vi "Configure Math.vi"(4 "dBm Resistance (600 Ohms)":i32(ring)=600 items=["50"=50, "75"=75, "93"=93, "110"=110, "124"=124, "125"=125, "135"=135, "150"=150, "250"=250, "300"=300, "500"=500, "600"=600, "800"=800, "900"=900, "1000"=1000, "1200"=1200, "8000"=8000], 5 "dB Reference (0.00 dBm)":dbl format="%.2f", 6 "Lower Limit (0.00)":dbl format="%.2f", 7 "Upper Limit (0.00)":dbl format="%.2f", 8 "error in (no error)":errorcluster, 9 "REL Offset (0.00)":dbl format="%_3f", 10 "Math Operation (0:None)":T1(ring), 11 "VISA resource name":refnum<visa-resource-name>) -> (0 "error out":errorcluster, 3 "VISA resource name out":refnum<visa-resource-name>)   [LabVIEW 2020, in "Library Instrument & Equipement.lvlib" / "Library Multimeter.lvlib" / "RIGOL DM3058.lvlib"]
doc: "Configures the Math Function on the instrument."
uses:
  RIGOL DM3058.lvlib
panel:
  # "Limit"
  # "DB Measurements"
  # "Offset"
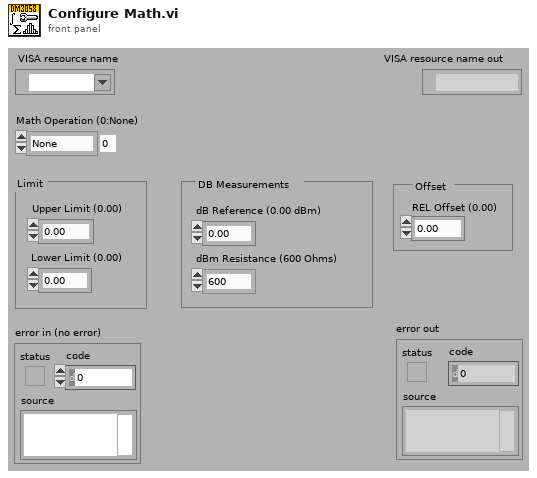
[diagram p1: front panel]
types:
  T1 = enum16{"None", "MAX", "MIN", "AVG", "P/F", "dB", "dBm", "REL"}
  T2 = cluster{"DM Series Mode":u16, "Measurement Function":u16}
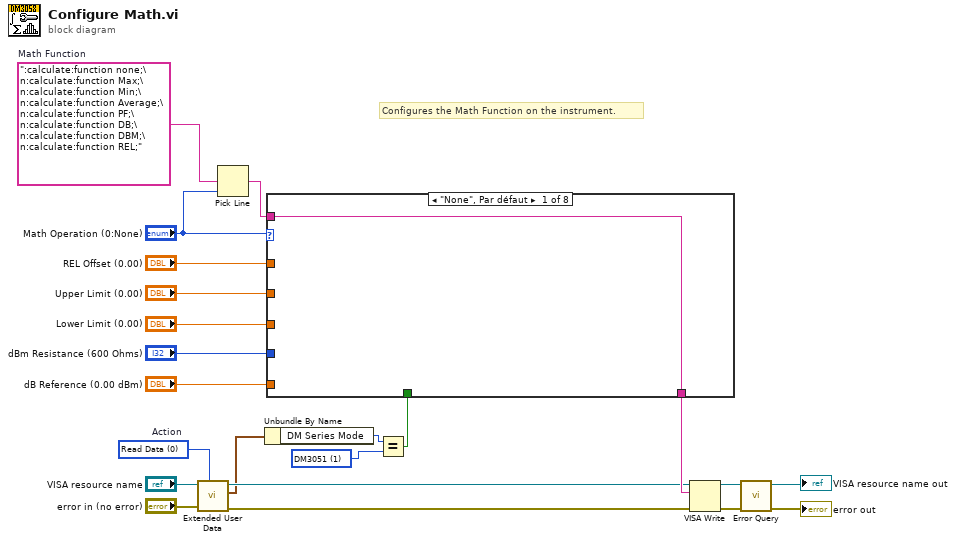
[diagram p0: block diagram]
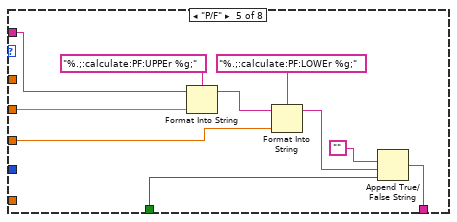
[diagram p5: hidden frame]
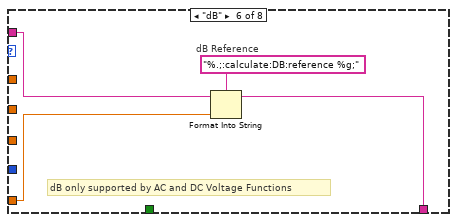
[diagram p6: hidden frame]
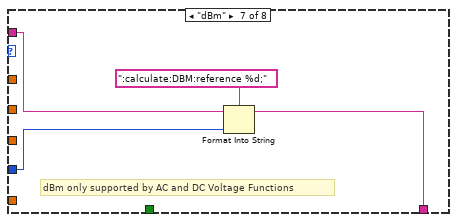
[diagram p7: hidden frame]
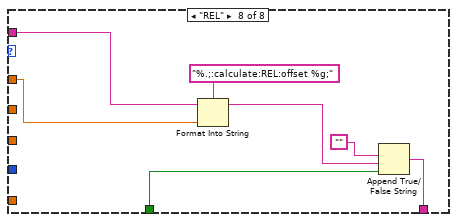
[diagram p8: hidden frame]
diagram:
  w4 = u16 1 items=["DM3058", "DM3051", "DM3068", "DM3058E"] ("DM Series Mode")
  w12 = 0 items=["Read Data", "Write Data", "Clear Data", "Clear ALL Data"]  # Action
  w22 = ":calculate:function none;\n:calculate:function Max;\n:calculate:function Min;\n:calculate:function Average;\n:calculate:function PF;\n:calculate:function DB;\n:calculate:function DBM;\n:calculate:function REL;"  # Math Function
  # "Configures the Math Function on the instrument."
  n1 = call "Extended User Data.vi"("Action (1: Write Data)"=w12, "Error In (no error)"="error in (no error)", "VISA resource name in"="VISA resource name") -> ("Error Out"=w13:errorcluster, "User Data Out"=w3:T2, "VISA resource name out"=w14:refnum<visa-resource-name>)  [unwired: 1 in, 5 out]
  n2 = Pick Line(multi-line string=w22, line index="Math Operation (0:None)") -> (output string=w21:string)  [unwired: 1 out]
  n3 = Unbundle By Name(w3) -> ("DM Series Mode"=w1:u16)
  n4 = Equal?(x=w1, y=w4) -> (x = y?=w2:bool)
  n5 = case shown="\"None\", Par défaut" "Math Operation (0:None)" {
    tunnel: w21 -> [w23 w24 w25 w26 w33 w40 w42 w50]
    tunnel: [w23 w24 w25 w26 w30 w38 w43 w48] -> w19
    tunnel: "Upper Limit (0.00)" -> [_ _ _ _ w32 _ _ _]
    tunnel: "Lower Limit (0.00)" -> [_ _ _ _ w31 _ _ _]
    tunnel: w2 -> [_ _ _ _ w29 _ _ w46]
    tunnel: "REL Offset (0.00)" -> [_ _ _ _ _ _ _ w45]
    tunnel: "dBm Resistance (600 Ohms)" -> [_ _ _ _ _ _ w41 _]
    tunnel: "dB Reference (0.00 dBm)" -> [_ _ _ _ _ w37 _ _]
    frame "None", Default {
    }
    frame "MAX" {
    }
    frame "MIN" {
    }
    frame "AVG" {
    }
    frame "P/F" {
      n6 = Format Into String(format string="%.;:calculate:PF:UPPEr %g;", initial string=w33, w32) -> (resulting string=w34:string)  [unwired: 1 in, 1 out]
      n7 = Format Into String(format string="%.;:calculate:PF:LOWEr %g;", initial string=w34, w31) -> (resulting string=w27:string)  [unwired: 1 in, 1 out]
      n8 = Append True/False String(1:w29, 2:w27, 3:"") -> (0:w30:string)  [unwired: 1 out]
    }
    frame "dB" {
      # "dB only supported by AC and DC Voltage Functions"
      # "dB Reference"
      n9 = Format Into String(format string="%.;:calculate:DB:reference %g;", initial string=w40, w37) -> (resulting string=w38:string)  [unwired: 1 in, 1 out]
    }
    frame "dBm" {
      # "dBm only supported by AC and DC Voltage Functions"
      n10 = Format Into String(format string=":calculate:DBM:reference %d;", initial string=w42, w41) -> (resulting string=w43:string)  [unwired: 1 in, 1 out]
    }
    frame "REL" {
      n11 = Format Into String(format string="%.;:calculate:REL:offset %g;", initial string=w50, w45) -> (resulting string=w47:string)  [unwired: 1 in, 1 out]
      n12 = Append True/False String(1:w46, 2:w47, 3:"") -> (0:w48:string)  [unwired: 1 out]
    }
  }
  n13 = VISA Write(VISA resource name=w14, write buffer=w19, error in (no error)=w13) -> (VISA resource name out=w8:refnum<visa-resource-name>, error out=w7:errorcluster)  [unwired: 1 out]
  n14 = call "Error Query.vi"("error in (no error)"=w7, "VISA resource name"=w8) -> ("error out"=→"error out":errorcluster, "VISA resource name out"=→"VISA resource name out":refnum<visa-resource-name>)  [unwired: 6 in, 2 out]
